vi "Redetection_Distribution.vi"(5 "Detected Event (1D) IN":cluster{dbl[][]}[](array[cluster]), 6 "Sweep trace (1D) IN":cluster{"Ramp Pattern":dbl[], "X":dbl[]}[](array[cluster]), 7 "Threshold":dbl, 8 "Detected event IN":cluster{dbl[][]}, 9 "New baseline info IN":cluster{dbl[][]}) -> (0 "EVT # (redetected)":i32, 1 "Sweep trace (1D) Out":cluster{"Ramp Pattern":dbl[], "X":dbl[]}[](array[cluster]), 2 "Averaged amplitude (pA)":dbl caption="평균" format="%0.2f", 3 "New baseline info OUT":cluster{dbl[][]}, 4 "Detected Event OUT":cluster{dbl[][]})   [LabVIEW 2017]
uses:
  <vilib>/Analysis/NI_AALBase.lvlib
panel:
  out "Whole trace":cluster{"Ramp Pattern":dbl[], "X":dbl[]}[](graph)
  out "크기":bool
  out "순서":bool
  in  "정지":bool
  out "event":cluster{dbl[], dbl[]}[](graph)
  in  "Event #":i16=4
  out "Distribution (output)":T1
  out "Event final OUT":dbl[][](array[numeric])
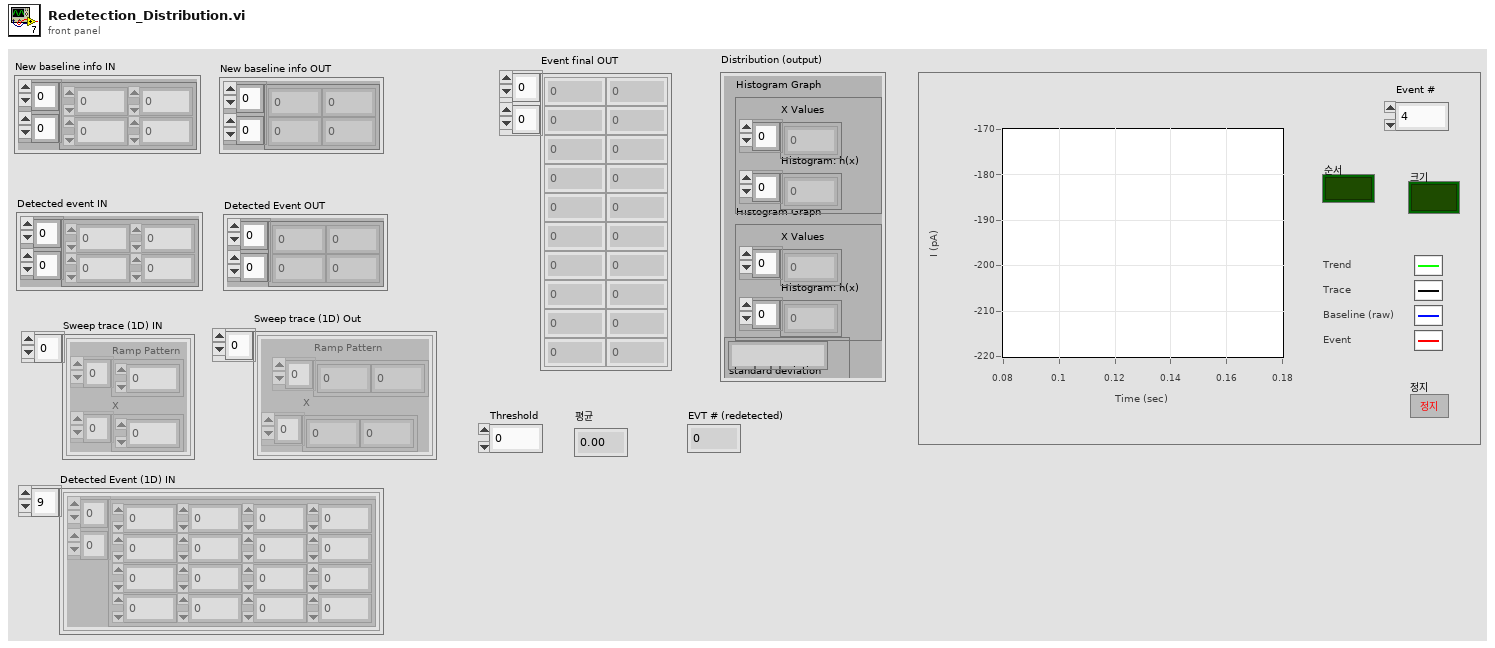
[diagram p1: front panel]
types:
  T1 = cluster{"Histogram Graph":cluster{"X Values":dbl[], "Histogram: h(x)":i32[]}, "Histogram Graph":cluster{"X Values":dbl[], "Histogram: h(x)":i32[]}, cluster{string, "standard deviation":string, "standard deviation":string}, i32[]}
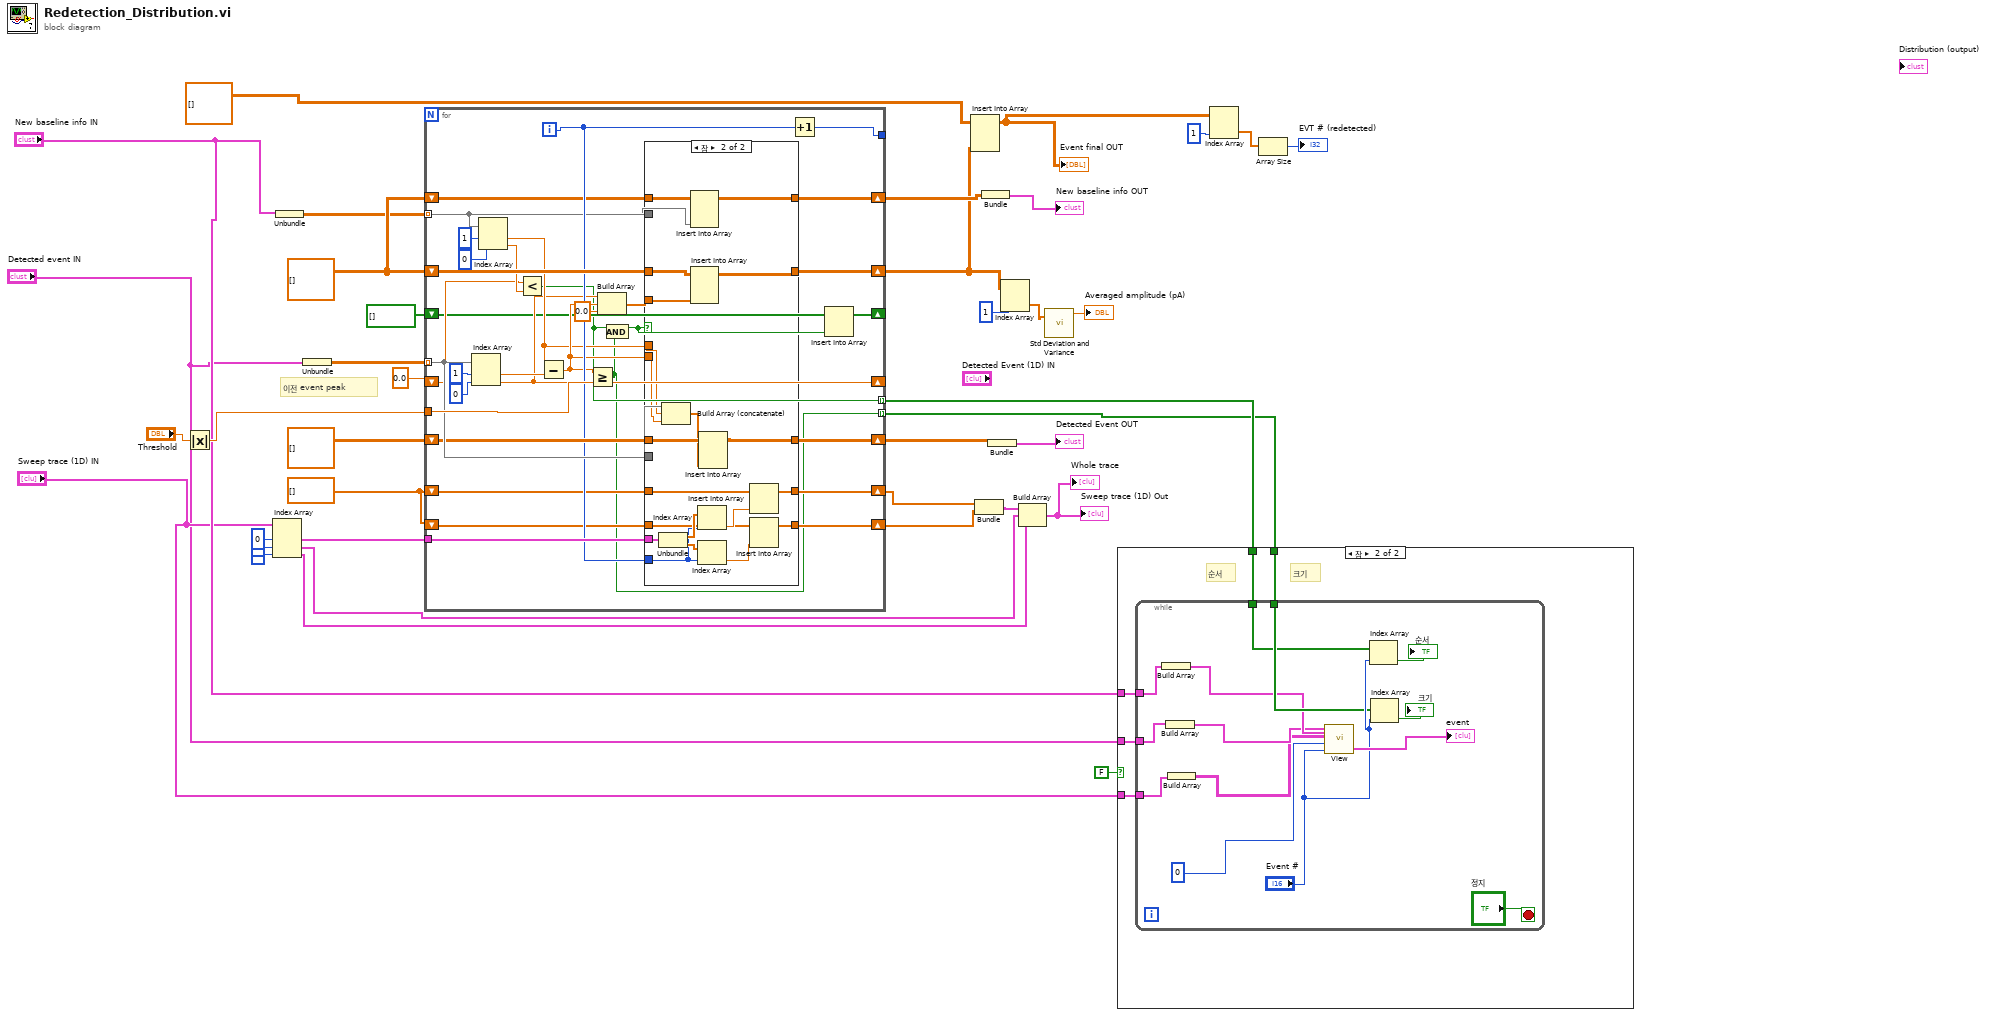
[diagram p0: block diagram]
diagram:
  w23 = dbl[] []
  w16 = dbl[][] []
  # "이전 event peak"
  n1 = Absolute Value(x="Threshold") -> (abs(x)=w34:dbl)
  n2 = Index Array(array="Sweep trace (1D) IN", index #1=0 ("인덱스"), index #2=1 ("인덱스"), index #3=2 ("인덱스")) -> (element #1=w24:cluster{"Ramp Pattern":dbl[], "X":dbl[]}, element #2=w18:cluster{"Ramp Pattern":dbl[], "X":dbl[]}, element #3=w17:cluster{"Ramp Pattern":dbl[], "X":dbl[]})
  n3 = Unbundle("New baseline info IN") -> (w8:dbl[][])
  n4 = Unbundle("Detected event IN") -> (w28:dbl[][])
  n5 = for {
    tunnel: w28 -> [w63] mode=indexing
    tunnel: [w65] -> _
    shift-right: [w67] -> w11
    shift-left: w16 -> [w66]
    tunnel: w34 -> [w64]
    shift-right: [w62] -> w26
    shift-left: dbl[][] [] -> [w61]
    tunnel: w24 -> [w59]
    shift-right: [w56] -> w14
    shift-left: w23 -> [w55]
    shift-right: [w57] -> w22
    shift-left: w23 -> [w54]
    tunnel: w8 -> [w51] mode=indexing
    shift-right: [w53] -> w15
    shift-left: w16 -> [w52]
    shift-right: [w46] -> _
    shift-left: 0.0 ("Numeric") -> [w44]
    shift-right: [w42] -> _
    shift-left: bool[] [] -> [w41]
    tunnel: [w40] -> w31 mode=indexing
    tunnel: [w39] -> w30 mode=indexing
    i -> [w58]
    n6 = Index Array(array=w63, index #1=1 ("인덱스"), index #2=0 ("인덱스")) -> (element #1=w70:dbl, element #2=w46:dbl)
    n7 = Index Array(array=w51, index #1=1 ("인덱스"), index #2=0 ("인덱스")) -> (element #1=w48:dbl, element #2=w45:dbl)
    n8 = Less?(x=w44, y=w45) -> (x < y?=w40:bool)
    n9 = Subtract(x=w48, y=w70) -> (x-y=w49:dbl)
    n10 = Greater Or Equal?(x=w49, y=w64) -> (x >= y?=w39:bool)
    n11 = Build Array(w46, w49, 0.0 ("원소")) -> (w68:dbl[])
    n12 = And(x=w40, y=w39) -> (x .and. y?=w43:bool)
    n13 = case shown="참" w43 {
      tunnel: w68 -> [_ w98]
      tunnel: [w76 w97] -> w67
      tunnel: w66 -> [w76 w96]
      tunnel: w63 -> [_ w80]
      tunnel: [w75 w95] -> w62
      tunnel: w61 -> [w75 w94]
      tunnel: w59 -> [_ w93]
      tunnel: w58 -> [_ w90]
      tunnel: [w73 w87] -> w57
      tunnel: [w74 w86] -> w56
      tunnel: w55 -> [w74 w85]
      tunnel: w54 -> [w73 w84]
      tunnel: w51 -> [_ w83]
      tunnel: [w72 w82] -> w53
      tunnel: w52 -> [w72 w81]
      tunnel: w49 -> [_ w78]
      tunnel: w48 -> [_ w79]
      frame False {
      }
      frame True {
        n14 = Unbundle(w93) -> ("Ramp Pattern"=w92:dbl[], "X"=w91:dbl[])
        n15 = Build Array (concatenate)(w80, w79, w78) -> (w77:dbl[])
        n16 = Insert Into Array(array=w81, new element=w83) -> (w82:dbl[][])  [unwired: 2 in]
        n17 = Insert Into Array(array=w96, new element=w98) -> (w97:dbl[][])  [unwired: 2 in]
        n18 = Index Array(array=w92, index=w90) -> (element=w89:dbl)
        n19 = Index Array(array=w91, index=w90) -> (element=w88:dbl)
        n20 = Insert Into Array(array=w94, new element=w77) -> (w95:dbl[][])  [unwired: 2 in]
        n21 = Insert Into Array(array=w85, new element=w89) -> (w86:dbl[])  [unwired: 1 in]
        n22 = Insert Into Array(array=w84, new element=w88) -> (w87:dbl[])  [unwired: 1 in]
      }
    }
    n23 = Increment(x=w58) -> (x+1=w65:i32)
    n24 = Insert Into Array(array=w41, new element=w43) -> (w42:bool[])  [unwired: 1 in]
  }
  n25 = Insert Into Array(array=dbl[][] [], new element=w11) -> (w36:dbl[][])  [unwired: 2 in]
  "Event final OUT" <- w36
  n26 = Bundle(w14, w22) -> (w21:cluster{dbl[], dbl[]})  [unwired: 1 in]
  n27 = Bundle(w15) -> (→"New baseline info OUT":cluster{dbl[][]})  [unwired: 1 in]
  n28 = Bundle(w26) -> (→"Detected Event OUT":cluster{dbl[][]})  [unwired: 1 in]
  n29 = Index Array(array=w11, index (col)=1 ("비활성화된 인덱스 (열)")) -> (element=w12:dbl[])  [unwired: 1 in]
  n30 = Build Array(w21, w18, w17) -> (→"Sweep trace (1D) Out" →"Whole trace":cluster{"Ramp Pattern":dbl[], "X":dbl[]}[])
  n31 = call <vilib>:"Std Deviation and Variance.vi"("X"=w12) -> ("mean"=→"Averaged amplitude (pA)":dbl)  [unwired: 1 in, 2 out]
  n32 = case shown="참" FALSE {
    tunnel: "New baseline info IN" -> [_ w103]
    tunnel: "Detected event IN" -> [_ w102]
    tunnel: "Sweep trace (1D) IN" -> [_ w101]
    tunnel: w31 -> [_ w100]
    tunnel: w30 -> [_ w99]
    frame False {
    }
    frame True {
      # "크기"
      # "순서"
      n33 = while {
        tunnel: w103 -> [w110]
        tunnel: w102 -> [w108]
        tunnel: w101 -> [w106]
        tunnel: w100 -> [w111]
        tunnel: w99 -> [w112]
        stop <- "정지" stop-if-true
        n34 = Build Array(w110) -> (w109:cluster{dbl[][]}[])
        n35 = Build Array(w108) -> (w107:cluster{dbl[][]}[])
        n36 = Build Array(w106) -> (w105:cluster{"Ramp Pattern":dbl[], "X":dbl[]}[][])
        n37 = call "View.vi"("Event #"="Event #", "Sweep #"=i16 0, "Baseline info new OUT"=w109, "Sweep trace (2D) In"=w105, "Detected Event (1D) In"=w107) -> ("event"=→"event":cluster{dbl[], dbl[]}[])  [unwired: 3 in, 2 out]
        n38 = Index Array(array=w111, index="Event #") -> (element=→"순서":bool)
        n39 = Index Array(array=w112, index="Event #") -> (element=→"크기":bool)
      }
    }
  }
  n40 = Index Array(array=w36, index (col)=1 ("비활성화된 인덱스 (열)")) -> (element=w2:dbl[])  [unwired: 1 in]
  n41 = Array Size(array=w2) -> (size(s)=→"EVT # (redetected)":i32)
